vi "Tektronix MSO5X Series Acquire Continuous Waveform.vi"() -> ()   [LabVIEW 2019]
doc: "Demonstrates how to set up an oscilloscope automatically. You can configure this VI to acquire waveforms continuously from a single channel by following the following steps:\n\n1. Specify a valid VISA resource to use. \n2. Specify a channel. \n3. Specify a time-out value for reading a waveform.\n4. Specifies the start and end point for reading a waveform.\n5. Run this VI. The <B>Waveform Graph</B> displays the waveform you acquire."
uses:
  <vilib>/Analysis/baseanly.llb/Mean (DBL).vi
  <instrlib>/Tektronix MSO5X Series/Public/Data/Read (Single Waveform).vi
  <instrlib>/Tektronix MSO5X Series/Tektronix MSO5X Series.lvlib
  <vilib>/Analysis/NI_AALBase.lvlib
panel:
  out "mean":dbl format="%0.6f"
  in  "Vertical Range (10.0 V)":dbl=10.0
  out "Waveform Graph":waveform(dbl)(graph)
  in  "Close Button":bool
  in  "Channel (CH1)":string="CH1"
  in  "Ending Point (2500)":i32=2500
  in  "Maximum Time (100000 ms)":u32=100000
  in  "VISA resource name":refnum<visa-resource-name>
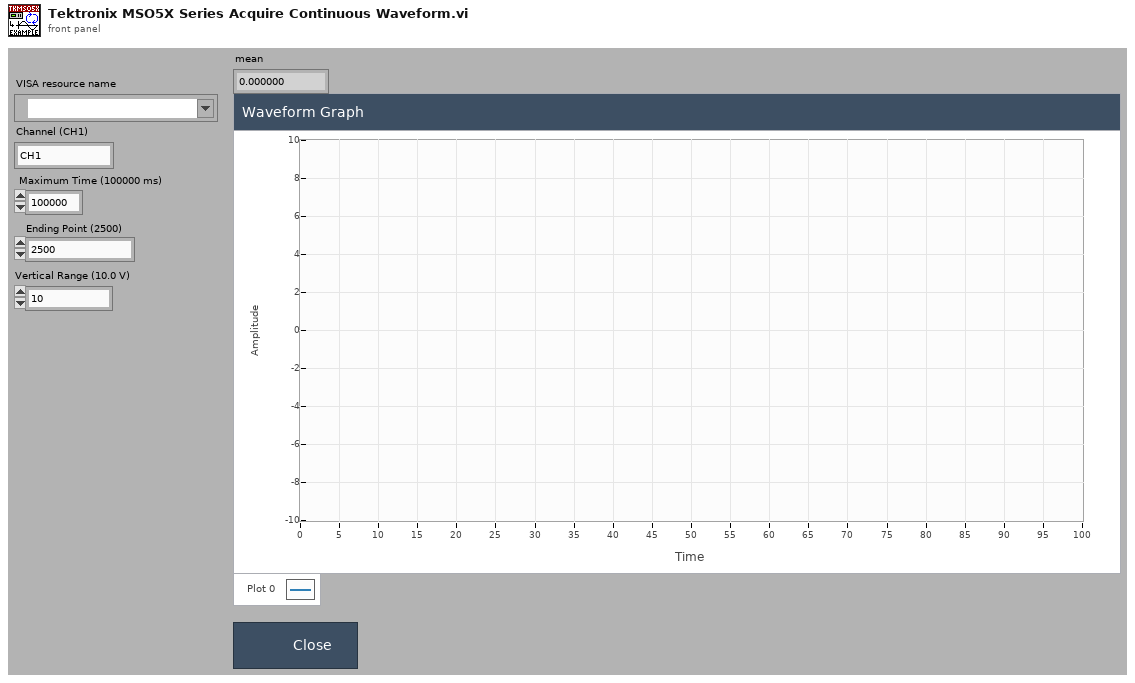
[diagram p1: front panel]
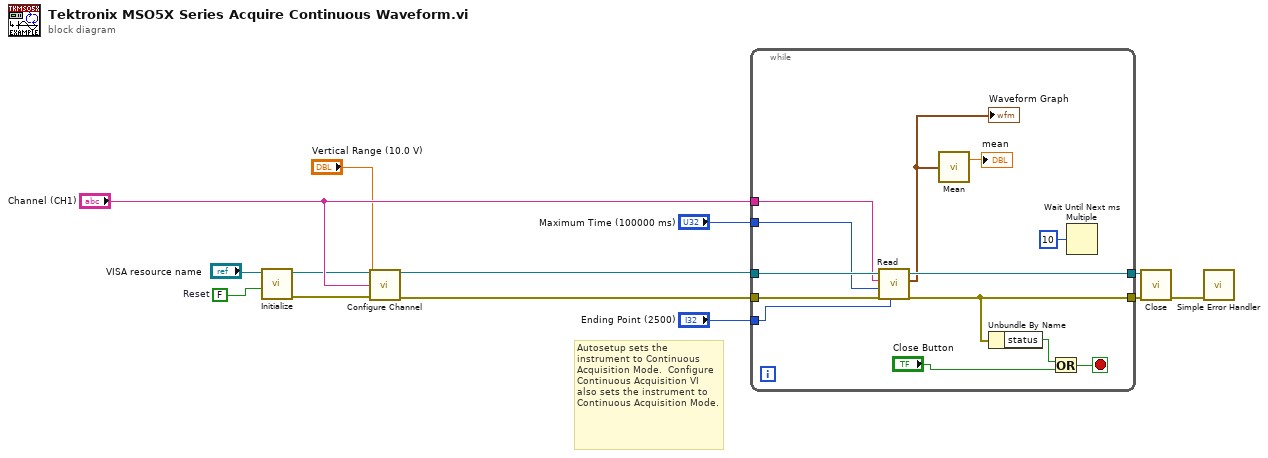
[diagram p0: block diagram]
diagram:
  w8 = FALSE  # Reset
  # "Autosetup sets the instrument to Continuous Acquisition Mode.  Configure Continuous Acquisition VI also sets the instrument to Continuous Acquisition Mode."
  n1 = call <instrlib>:"Initialize.vi"("Reset (True)"=w8, "VISA resource name"="VISA resource name") -> ("error out"=w5:errorcluster, "VISA resource name out"=w4:refnum<visa-resource-name>)  [unwired: 8 in]
  n2 = call <instrlib>:"Configure Channel.vi"("VISA resource name"=w4, "Channel (CH1)"="Channel (CH1)", "Vertical Range (10.0 V)"="Vertical Range (10.0 V)", "error in (no error)"=w5) -> ("VISA resource name out"=w3:refnum<visa-resource-name>, "error out"=w2:errorcluster)  [unwired: 10 in]
  n3 = while {
    tunnel: w3 -> [w21]
    tunnel: w2 -> [w20]
    tunnel: [w22] -> w13
    tunnel: [w23] -> w12
    tunnel: "Maximum Time (100000 ms)" -> [w19]
    tunnel: "Ending Point (2500)" -> [w18]
    tunnel: "Channel (CH1)" -> [w17]
    stop <- w24 stop-if-true
    n4 = call-poly <instrlib>:"Read.vi"("Ending Point (2500)"=w18, "error in (no error)"=w20, "Maximum Time (100000 ms)"=w19, "Channel (CH1)"=w17, "VISA resource name"=w21) -> ("error out"=w23:errorcluster, "Waveform Graph"=w15:waveform(dbl), "VISA resource name out"=w22:refnum<visa-resource-name>)  [unwired: 4 in]
    "Waveform Graph" <- w15
    n5 = call-poly <vilib>:"Mean.vi"("X"=w15) -> ("mean"=→"mean":dbl)  [unwired: 1 out]
    n6 = Unbundle By Name(w23) -> ("status"=w25:bool)
    n7 = Or(x=w25, y="Close Button") -> (x .or. y?=w24:bool)
    n8 = Wait Until Next ms Multiple(millisecond multiple=u32 10) -> ()  [unwired: 1 out]
  }
  n9 = call <instrlib>:"Close.vi"("error in (no error)"=w12, "VISA resource name"=w13) -> ("error out"=w11:errorcluster)  [unwired: 9 in]
  n10 = call <vilib>:"Simple Error Handler.vi"("error in (no error)"=w11) -> ()  [unwired: 4 in, 5 out]
